vi "HJ212-2005.vi"(8 "error in (no error)":errorcluster caption="错误输入（无错误）", 11 "数据块":T1) -> (0 "error out":errorcluster caption="错误输出", 2 "通讯包字符串":string, 3 "通讯包":T2={"包头"="##", "数据段长度"="", "数据段"="", "CRC"="", "包尾"="\r\n"})   [LabVIEW 2016, in "数据传输系统-03.lvlib"]
panel:
  # "范例代码：\n\n##0101QN=20160801085857223;ST=32;CN=1062;PW=100000;MN=010000A8900016F000169DC0;Flag=5\n;CP=&&RtdInterval=30&&1C80\\r\\n"
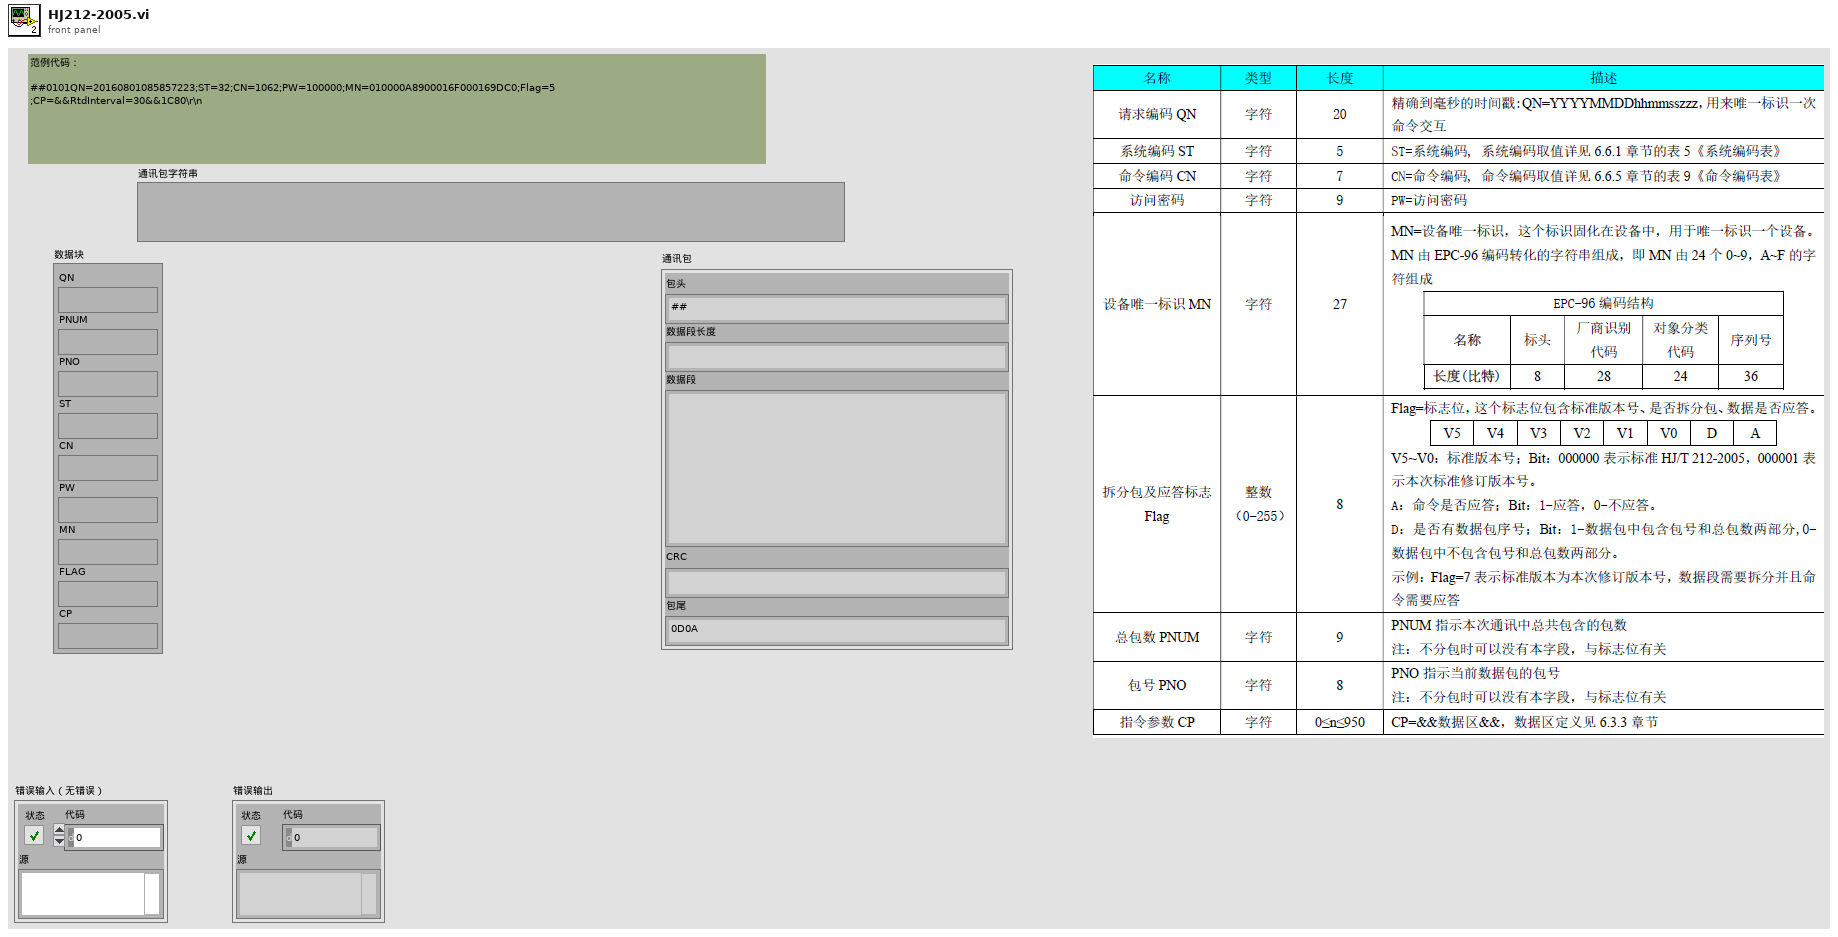
[diagram p1: front panel]
types:
  T1 = cluster{"QN":string, "ST":string, "CN":string, "PW":string, "MN":string, "FLAG":string, "PNUM":string, "PNO":string, "CP":string}
  T2 = cluster{"包头":string, "数据段长度":string, "数据段":string, "CRC":string, "包尾":string}
  T3 = cluster{"QN":string, "PNUM":string, "PNO":string, "ST":string, "CN":string, "PW":string, "MN":string, "FLAG":string, "CP":string}
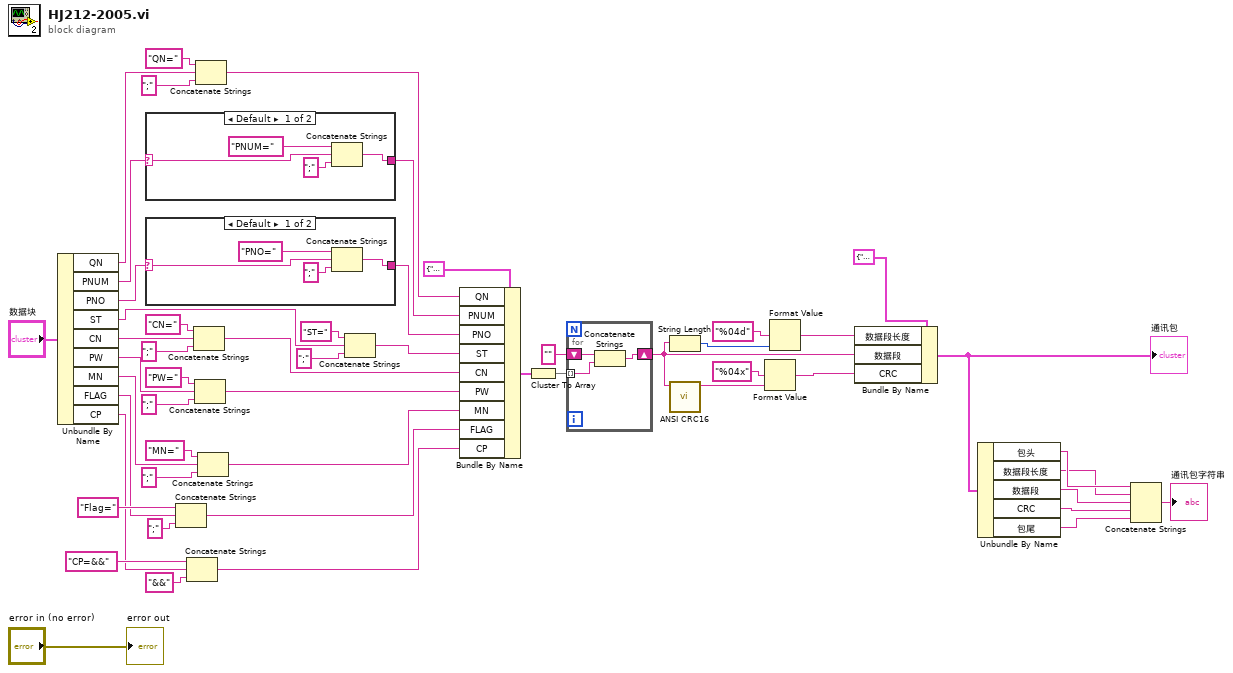
[diagram p0: block diagram]
diagram:
  n1 = Unbundle By Name("数据块") -> ("QN"=w17:string, "PNUM"=w16:string, "PNO"=w15:string, "ST"=w14:string, "CN"=w13:string, "PW"=w12:string, "MN"=w11:string, "FLAG"=w10:string, "CP"=w9:string)
  n2 = case shown="Default" w16 {
    selector: w16 -> [w55 w58]
    tunnel: [w54 w58] -> w27
    frame Default {
      n3 = Concatenate Strings("PNUM=" ("字符串"), w55, ";" ("字符串")) -> (w54:string)
    }
    frame "" {
    }
  }
  n4 = case shown="Default" w15 {
    selector: w15 -> [w60 w63]
    tunnel: [w59 w63] -> w26
    frame Default {
      n5 = Concatenate Strings("PNO=" ("字符串"), w60, ";" ("字符串")) -> (w59:string)
    }
    frame "" {
    }
  }
  n6 = Concatenate Strings("Flag=" ("字符串"), w10, ";" ("字符串")) -> (w21:string)
  n7 = Concatenate Strings("CP=&&" ("字符串"), w9, "&&" ("字符串")) -> (w20:string)
  n8 = Concatenate Strings("CN=" ("字符串"), w13, ";" ("字符串")) -> (w24:string)
  n9 = Concatenate Strings("PW=" ("字符串"), w12, ";" ("字符串")) -> (w23:string)
  n10 = Concatenate Strings("QN=" ("字符串"), w17, ";" ("字符串")) -> (w28:string)
  n11 = Concatenate Strings("MN=" ("字符串"), w11, ";" ("字符串")) -> (w22:string)
  n12 = Concatenate Strings("ST=" ("字符串"), w14, ";" ("字符串")) -> (w25:string)
  n13 = Bundle By Name(cluster=T3 {"QN"="", "PNUM"="", "PNO"="", "ST"="", "CN"="", "PW"="", "MN"="", "FLAG"="", "CP"=""} ("数据段"), "QN"=w28, "PNUM"=w27, "PNO"=w26, "ST"=w25, "CN"=w24, "PW"=w23, "MN"=w22, "FLAG"=w21, "CP"=w20) -> (w19:T3)
  n14 = Cluster To Array(cluster=w19) -> (array=w50:string[])
  n15 = for {
    tunnel: w50 -> [w64] mode=indexing
    shift-right: [w65] -> w44
    shift-left: "" ("QN") -> [w66]
    n16 = Concatenate Strings(w66, w64) -> (w65:string)
  }
  n17 = String Length(string=w44) -> (length=w48:i32)
  n18 = call "ANSI CRC16.vi"("puchMsg"=w44) -> ("数据段长度"=w45:string)  [unwired: 8 in, 2 out]
  n19 = Format Value(format string="%04x" ("格式字符串"), value (0)=w45) -> (output string=w47:string)  [unwired: 1 in]
  n20 = Format Value(format string="%04d" ("格式字符串"), value (0)=w48) -> (output string=w51:string)  [unwired: 1 in]
  n21 = Bundle By Name(cluster=T2 {"包头"="##", "数据段长度"="", "数据段"="", "CRC"="", "包尾"="\r\n"} ("通讯包"), "数据段长度"=w51, "数据段"=w44, "CRC"=w47) -> (w7:T2)
  "通讯包" <- w7
  n22 = Unbundle By Name(w7) -> ("包头"=w6:string, "数据段长度"=w5:string, "数据段"=w4:string, "CRC"=w3:string, "包尾"=w2:string)
  n23 = Concatenate Strings(w6, w5, w4, w3, w2) -> (→"通讯包字符串":string)
  "error out" <- "error in (no error)"
